vi "Random_Numbers.vi"() -> ()   [LabVIEW 2024]
panel:
  out "Array":dbl[](array[numeric])
  in  "Numeric":i32
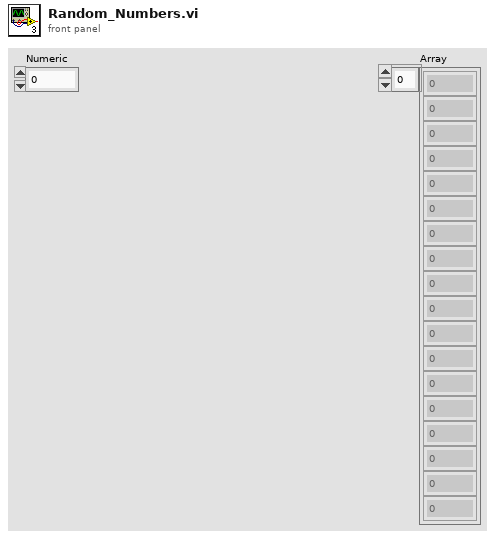
[diagram p1: front panel]
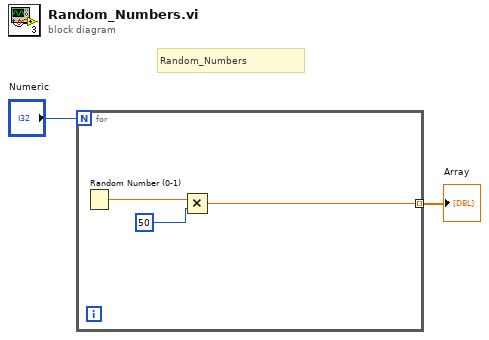
[diagram p0: block diagram]
diagram:
  # "Random_Numbers"
  n1 = for {
    N: "Numeric" -> [_]
    tunnel: [w3] -> w1 mode=indexing
    n2 = Random Number (0-1)() -> (number: 0 to 1=w5:dbl)
    n3 = Multiply(x=w5, y=50) -> (x*y=w3:dbl)
  }
  "Array" <- w1
